vi "Append Data DBL.vi"(4 "transpose? (no:F)":bool=TRUE, 6 "append to file? (new file:F)":bool, 7 "format (%.3f)":string="%.6e", 8 "error in (no error)":errorcluster, 9 "Data":dbl[][](array[numeric]), 10 "Save data details":T1={"Data file path"=path "", "Comments file path"=path "", "Channel names"=["Frequency", "Signal_X", "Signal_Y", "IF_X", "IF_Y"]}, 11 "Save data settings":T2={"Save data"=TRUE, "Data Root Path"=path "", "File Prefix"="", "File Format"=enum."ASCII", "Save column names"=TRUE, "File Comments"="<Description of the current file>", "User/Prj"="<User Name/Project Description>"}) -> (0 "error out":errorcluster, 2 "Save data details out":T1)   [LabVIEW 2015]
uses:
  Controls/Save data settings.ctl
  Controls/File formats.ctl
  Controls/Save data details.ctl
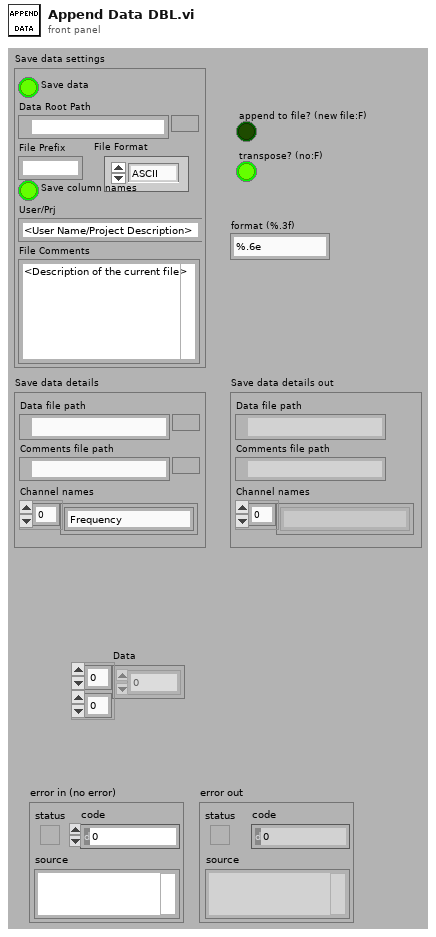
[diagram p1: front panel]
types:
  T1 = typedef "Save data details.ctl" = cluster{"Data file path":path, "Comments file path":path, "Channel names":string[]}
  T2 = typedef "Save data settings.ctl" = cluster{"Save data":bool, "Data Root Path":path, "File Prefix":string, "File Format":T3, "Save column names":bool, "File Comments":string, "User/Prj":string}
  T3 = typedef "File formats.ctl" = enum16{"TDMS", "ASCII", "BINARY"}
  T4 = enum16{"open", "open or create", "create or replace", "create", "open (read-only)"}
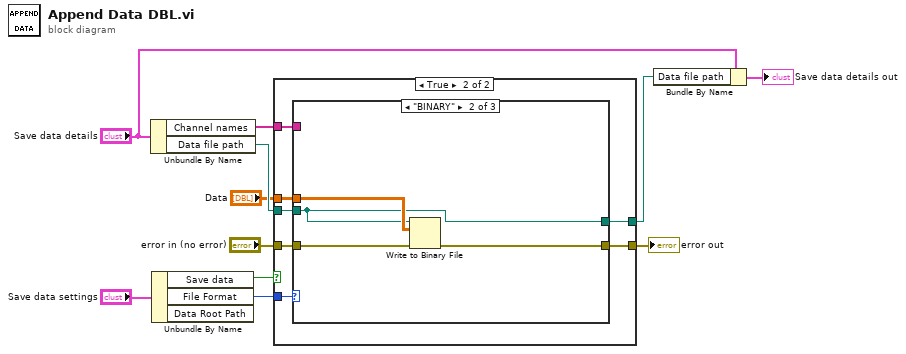
[diagram p0: block diagram]
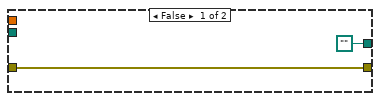
[diagram p2: hidden frame]
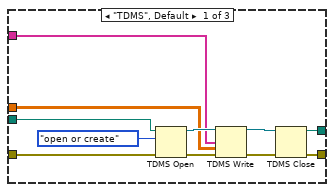
[diagram p3: hidden frame]
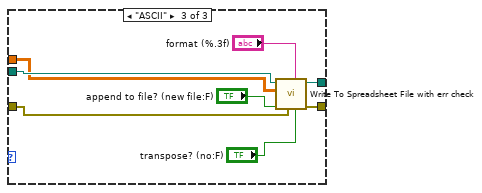
[diagram p4: hidden frame]
diagram:
  n1 = Unbundle By Name("Save data details") -> ("Channel names"=w4:string[], "Data file path"=w6:path)
  n2 = Unbundle By Name("Save data settings") -> ("Save data"=w8:bool, "File Format"=w11:T3)  [unwired: 1 out]
  n3 = case shown="True" w8 {
    tunnel: w11 -> [_ w20]
    tunnel: [path "" w19] -> w2
    tunnel: [w13 w18] -> w10
    tunnel: "error in (no error)" -> [w13 w17]
    tunnel: "Data" -> [_ w16]
    tunnel: w6 -> [_ w15]
    tunnel: w4 -> [_ w14]
    frame False {
    }
    frame True {
      n4 = case shown="\"BINARY\"" w20 {
        tunnel: w17 -> [w23 w35 w41]
        tunnel: [w22 w34 w40] -> w18
        tunnel: w15 -> [w30 w32 w39]
        tunnel: [w24 w32 w37] -> w19
        tunnel: w16 -> [w27 w33 w36]
        tunnel: w14 -> [w21 _ _]
        frame "TDMS", Default {
          n5 = TDMS Open(8:w23, 10:T4."open or create" ("operation (0:open)"), 11:w30) -> (0:w29:errorcluster, 3:w28:refnum<k34>)  [unwired: 4 in]
          n6 = TDMS Write(0:w28, 7:w21, 9:w27, 11:w29) -> (4:w25:refnum<k34>, 15:w26:errorcluster)  [unwired: 2 in, 2 out]
          n7 = TDMS Close(8:w26, 11:w25) -> (0:w22:errorcluster, 3:w24:path)
        }
        frame "BINARY" {
          n8 = Write to Binary File(file (use dialog)=w32, data=w33, error in=w35) -> (error out=w34:errorcluster)  [unwired: 3 in, 2 out]
        }
        frame "ASCII" {
          n9 = call "Write To Spreadsheet File with err check.vi"("transpose? (no:F)"="transpose? (no:F)", "format (%.3f)"="format (%.3f)", "error in (no error)"=w41, "append to file? (new file:F)"="append to file? (new file:F)", "2D data"=w36, "file path (dialog if empty)"=w39) -> ("error out"=w40:errorcluster, "new file path (Not A Path if cancelled)"=w37:path)  [unwired: 2 in, 2 out]
        }
      }
    }
  }
  "error out" <- w10
  n10 = Bundle By Name(cluster="Save data details", "Data file path"=w2) -> (→"Save data details out":T1)
